vi "add to memory format.vi"(8 "error in":errorcluster, 9 "NISE_CEF_serializable configuration in":refnum<class "NISE_CEF_serializable configuration.lvclass">, 10 "parent ID":string, 11 "memory hierarchy in":T1) -> (0 "error out":errorcluster, 3 "memory hierarchy out":T1)   [LabVIEW 2013, in "NISE_CEF_TreeSerializer.lvlib"]
uses:
  NISE_CEF_TreeSerializer.lvlib
  memory hierarchy.ctl
  hierarchy element.ctl
  serializable configuration/NISE_CEF_serializable configuration.lvclass
  serializable configuration/NISE_CEF_serializable configuration.lvclass/NISE_CEF_serializable configuration.ctl
  NISE_CEF_TreeControl.lvlib
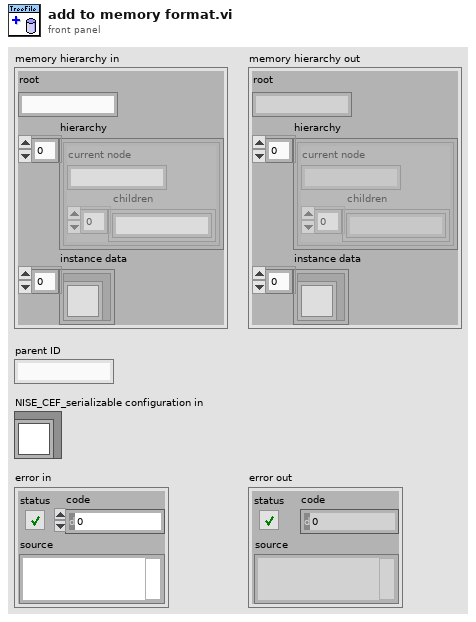
[diagram p1: front panel]
types:
  T1 = typedef "NISE_CEF_TreeSerializer.lvlib/memory hierarchy.ctl" = cluster{"root":string, "hierarchy":T2[], "instance data":refnum<class "NISE_CEF_serializable configuration.lvclass">[]}
  T2 = typedef "NISE_CEF_TreeSerializer.lvlib/hierarchy element.ctl" = cluster{"current node":string, "children":string[]}
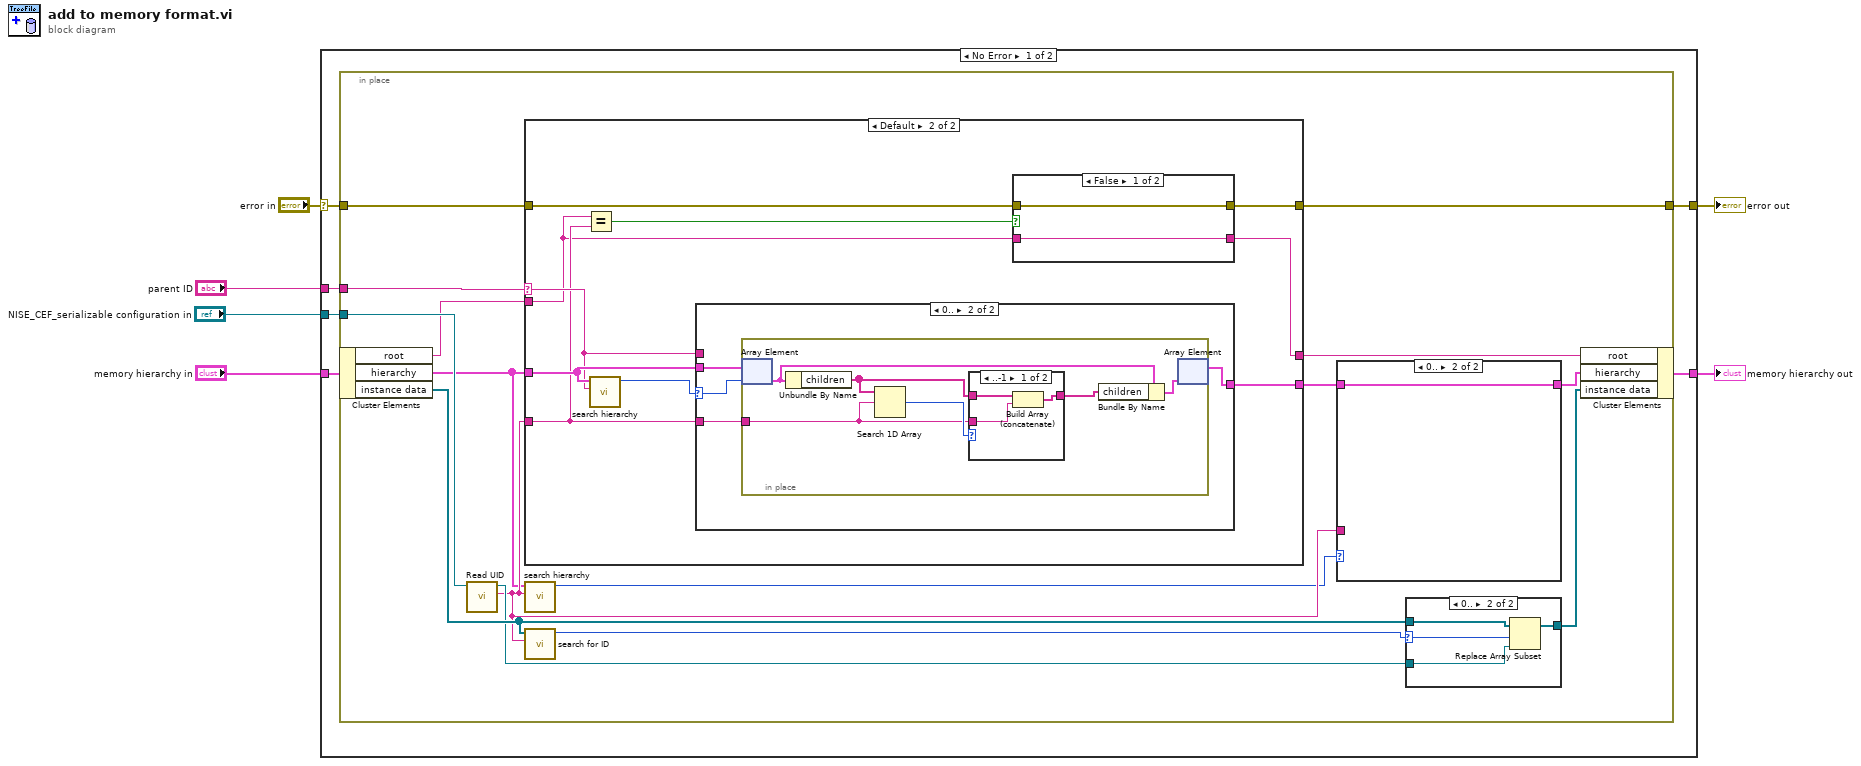
[diagram p0: block diagram]
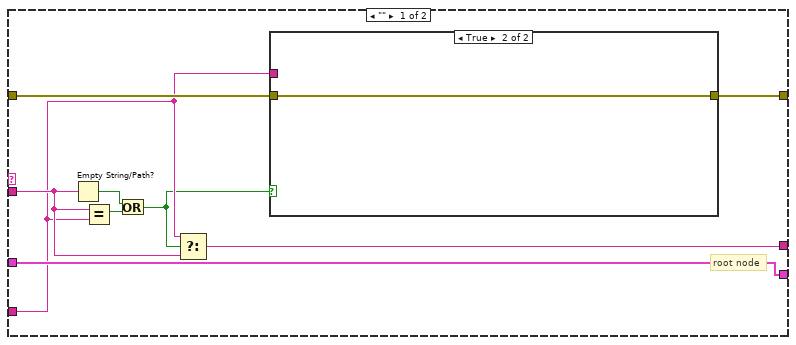
[diagram p2: hidden frame]
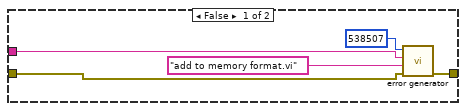
[diagram p3: hidden frame]
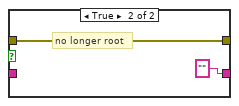
[diagram p4: hidden frame]
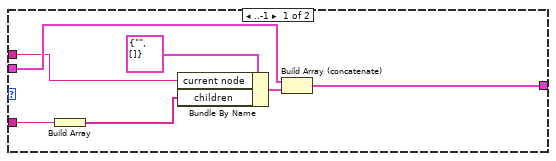
[diagram p5: hidden frame]
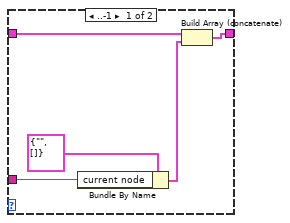
[diagram p7: hidden frame]
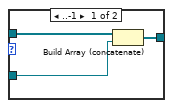
[diagram p8: hidden frame]
diagram:
  n1 = case shown="No Error" "error in" {
    selector: "error in" -> [w8 w92]
    tunnel: [w12 w91] -> w6
    tunnel: "memory hierarchy in" -> [w11 w91]
    tunnel: "parent ID" -> [w10 _]
    tunnel: "NISE_CEF_serializable configuration in" -> [w9 _]
    tunnel: [w7 w92] -> w1
    frame No Error {
      n2 = in-place {
        in-place-border: w9 -> [w27]
        in-place-border: w10 -> [w21]
        in-place-border: w8 -> [w15]
        in-place-border: [w14] -> w7
        n3 = in-place-cluster #1(w11) -> ("root"=w20:string, "hierarchy"=w17:T2[], "instance data"=w25:refnum<class "NISE_CEF_serializable configuration.lvclass">[])
        n4 = call "Read UID.vi"("configuration in"=w27) -> ("instance id"=w18:string, "configuration out"=w24:refnum<class "NISE_CEF_serializable configuration.lvclass">)  [unwired: 8 in, 1 out]
        n5 = case shown="Default" w21 {
          selector: w21 -> [_ w50]
          tunnel: w17 -> [w36 w51]
          tunnel: [w36 w52] -> w23
          tunnel: w18 -> [w29 w49]
          tunnel: w20 -> [w30 w46]
          tunnel: [w35 w47] -> w19
          tunnel: w15 -> [w34 w44]
          tunnel: [w33 w45] -> w14
          frame "" {
            # "root node"
            n6 = Empty String/Path?(string/path=w30) -> (empty?=w31:bool)
            n7 = Equal?(x=w30, y=w29) -> (x = y?=w32:bool)
            n8 = Or(x=w31, y=w32) -> (x .or. y?=w28:bool)
            n9 = Select(t=w29, s=w28, f=w30) -> (s? t:f=w35:string)
            n10 = case shown="True" w28 {
              tunnel: w34 -> [w41 w42]
              tunnel: [w40 w42] -> w33
              tunnel: w29 -> [w38 _]
              frame False {
                n11 = call "error generator.vi"("error in"=w41, "source"="add to memory format.vi", "append error message"=w38, "error code (0)"=538507) -> ("error out"=w40:errorcluster)  [unwired: 5 in]
              }
              frame True {
              }
            }
          }
          frame Default {
            n12 = Equal?(x=w46, y=w49) -> (x = y?=w48:bool)
            n13 = call "search hierarchy.vi"("ID"=w50, "hierarchy"=w51) -> ("index"=w43:i32)  [unwired: 9 in]
            n14 = case shown="0.." w43 {
              selector: w43 -> [_ w64]
              tunnel: w51 -> [w61 w67]
              tunnel: [w58 w66] -> w52
              tunnel: w49 -> [w60 w65]
              tunnel: w50 -> [w57 _]
              frame ..-1 {
                n15 = Build Array(w60) -> (w59:string[])
                n16 = Bundle By Name(cluster=T2 {"current node"="", "children"=[]} ("hierarchy"), "current node"=w57, "children"=w59) -> (w63:T2)
                n17 = Build Array (concatenate)(w61, w63) -> (w58:T2[])
              }
              frame 0.. {
                n18 = in-place {
                  in-place-border: w65 -> [w69]
                  n19 = in-place-array #2(w67, w64) -> (w73:T2)
                  n20 = Unbundle By Name(w73) -> ("children"=w70:string[])
                  n21 = Search 1D Array(1D array=w70, element=w69) -> (index of element=w71:i32)  [unwired: 1 in]
                  n22 = case shown="..-1" w71 {
                    tunnel: w70 -> [w76 w77]
                    tunnel: w69 -> [w75 _]
                    tunnel: [w74 w77] -> w68
                    frame ..-1 {
                      n23 = Build Array (concatenate)(w76, w75) -> (w74:string[])
                    }
                    frame 0.. {
                    }
                  }
                  n24 = Bundle By Name(cluster=w73, "children"=w68) -> (w72:T2)
                  n25 = in-place-array #2(w72) -> (w66:T2[])  [unwired: 1 out]
                }
              }
            }
            n26 = case shown="False" w48 {
              tunnel: [w54 "" ("root")] -> w47
              tunnel: w46 -> [w54 _]
              tunnel: [w53 w56] -> w45
              tunnel: w44 -> [w53 w56]
              frame False {
              }
              frame True {
                # "no longer root"
              }
            }
          }
        }
        n27 = call "search hierarchy.vi"("ID"=w18, "hierarchy"=w17) -> ("index"=w13:i32)  [unwired: 9 in]
        n28 = call "search for ID.vi"("instance id"=w18, "instance data"=w25) -> ("index"=w16:i32)  [unwired: 9 in]
        n29 = case shown="0.." w13 {
          tunnel: w23 -> [w82 w83]
          tunnel: [w81 w83] -> w22
          tunnel: w18 -> [w79 _]
          frame ..-1 {
            n30 = Bundle By Name(cluster=T2 {"current node"="", "children"=[]} ("hierarchy"), "current node"=w79) -> (w78:T2)
            n31 = Build Array (concatenate)(w82, w78) -> (w81:T2[])
          }
          frame 0.. {
          }
        }
        n32 = case shown="0.." w16 {
          selector: w16 -> [_ w87]
          tunnel: [w85 w89] -> w26
          tunnel: w25 -> [w84 w90]
          tunnel: w24 -> [w86 w88]
          frame ..-1 {
            n33 = Build Array (concatenate)(w84, w86) -> (w85:refnum<class "NISE_CEF_serializable configuration.lvclass">[])
          }
          frame 0.. {
            n34 = Replace Array Subset(array=w90, new element=w88, index=w87) -> (w89:refnum<class "NISE_CEF_serializable configuration.lvclass">[])
          }
        }
        n35 = in-place-cluster #1("root"=w19, "hierarchy"=w22, "instance data"=w26) -> (w12:T1)
      }
    }
    frame Error {
    }
  }
  "memory hierarchy out" <- w6
  "error out" <- w1
